vi "ASGS_device_serial_mode.vi"() -> ()   [LabVIEW 2017]
uses:
  <vilib>/Utility/file.llb/Read Delimited Spreadsheet (DBL).vi
  <vilib>/Instr/_visa.llb/VISA Configure Serial Port (Instr).vi
panel:
  in  "Match Pressure":bool
  out "While loop":dbl
  in  "Flow C. Baud Rate":u32=9600
  in  "Flow Controller Port":refnum<visa-resource-name>
  out "Constriction Percent":dbl
  out "Desired Subglottal Pressure":dbl
  in  "Number of Tests":dbl
  in  "SGS Device Port":refnum<visa-resource-name>
  in  "SGS Device Baud Rate":u32=9600
  out "Current Constriction":dbl
  # "SGS DEVICE CONTROL"
  # "USB Control"
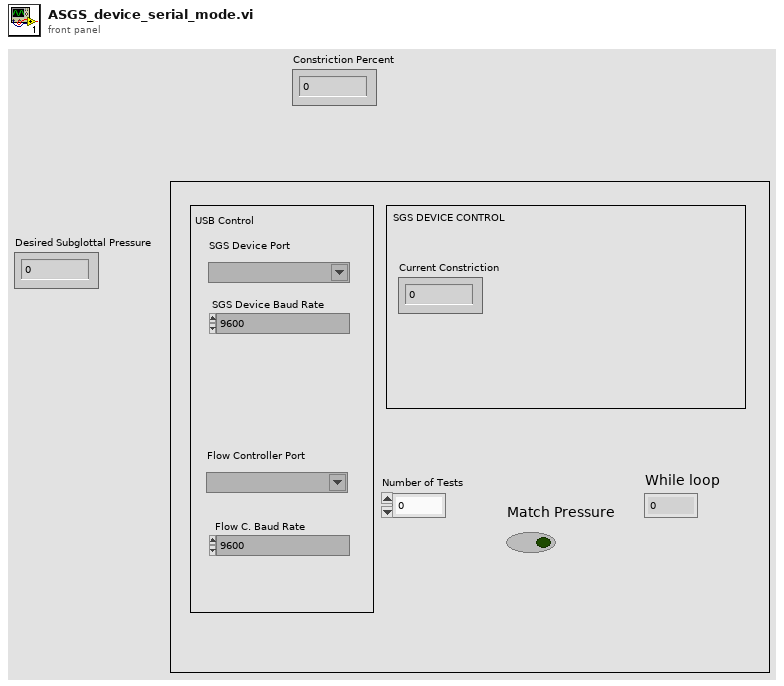
[diagram p1: front panel]
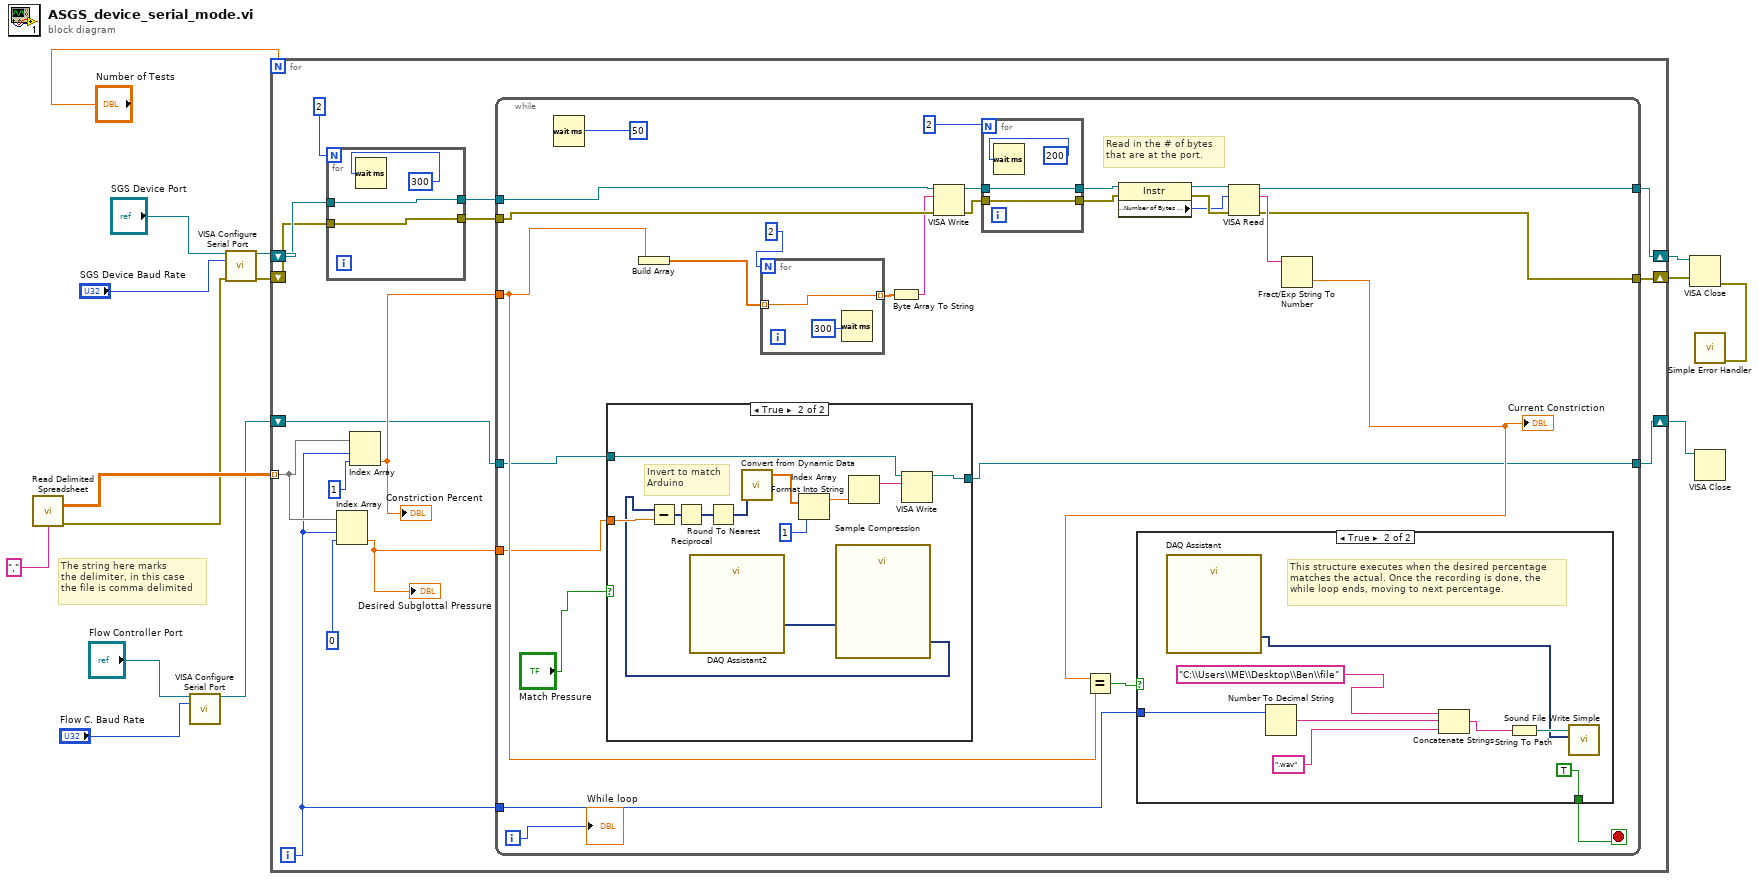
[diagram p0: block diagram]
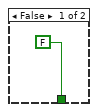
[diagram p3: hidden frame]
diagram:
  # "The string here marks\nthe delimiter, in this case\nthe file is comma delimited"
  n1 = call-poly <vilib>:"Read Delimited Spreadsheet.vi"("delimiter (\\t)"=",") -> ("all rows"=w8:dbl[][], "error out"=w6:errorcluster)  [unwired: 9 in, 4 out]
  n2 = call-poly "VISA Configure Serial Port"("VISA resource name"="Flow Controller Port", "baud rate (9600)"="Flow C. Baud Rate") -> ("VISA resource name out"=w2:refnum<visa-resource-name>)  [unwired: 12 in, 1 out]
  n3 = call-poly "VISA Configure Serial Port"("VISA resource name"="SGS Device Port", "baud rate (9600)"="SGS Device Baud Rate", "error in (no error)"=w6) -> ("VISA resource name out"=w10:refnum<visa-resource-name>, "error out"=w9:errorcluster)  [unwired: 11 in]
  n4 = for {
    N: "Number of Tests" -> [_]
    shift-right: [w23] -> w14
    shift-left: w10 -> [w20]
    shift-right: [w24] -> w15
    shift-left: w9 -> [w19]
    tunnel: w8 -> [w30] mode=indexing
    shift-right: [w22] -> w1
    shift-left: w2 -> [w25]
    i -> [w26]
    n5 = for {
      N: 2 -> [_]
      tunnel: [w33] -> w21
      tunnel: w20 -> [w33]
      tunnel: w19 -> [w32]
      tunnel: [w32] -> w18
      n6 = Wait (ms)(milliseconds to wait=300) -> ()  [unwired: 1 out]
    }
    n7 = Index Array(array=w30, index #1=w26, index #2=0) -> (element #2=w16:dbl)  [unwired: 1 out]
    "Desired Subglottal Pressure" <- w16
    n8 = Index Array(array=w30, index #1=w26, index #2=1) -> (element #2=w27:dbl)  [unwired: 1 out]
    "Constriction Percent" <- w27
    n9 = while {
      tunnel: w27 -> [w58]
      tunnel: w26 -> [w60]
      tunnel: w21 -> [w52]
      tunnel: w18 -> [w53]
      tunnel: [w48] -> w24
      tunnel: w25 -> [w37]
      tunnel: [w36] -> w22
      tunnel: [w47] -> w23
      tunnel: w16 -> [w35]
      i -> [w55]
      stop <- w56 stop-if-true
      # "Read in the # of bytes \nthat are at the port."
      n10 = Wait (ms)(milliseconds to wait=u32 50 ("millisecond timer value")) -> ()  [unwired: 1 out]
      n11 = case shown="True" "Match Pressure" {
        tunnel: w35 -> [_ w69]
        tunnel: [w62 w67] -> w36
        tunnel: w37 -> [w62 w66]
        frame False {
        }
        frame True {
          # "Invert to match\nArduino"
          n12 = call "DAQ Assistant2"() -> ("data"=w74:dynamicdata)  [unwired: 17 in, 2 out]
          n13 = call "Sample Compression"("Signals"=w74) -> ("Mean"=w68:dynamicdata)  [unwired: 8 in, 2 out]
          n14 = Subtract(x=w68, y=w69) -> (x-y=w65:dynamicdata)
          n15 = Reciprocal(x=w65) -> (1/x=w64:dynamicdata)
          n16 = Round To Nearest(number=w64) -> (nearest integer value=w63:dynamicdata)
          n17 = call "Convert from Dynamic Data"("Dynamic Data Type"=w63) -> ("Array"=w71:dbl[])  [unwired: 3 in]
          n18 = Index Array(array=w71, index=1) -> (element=w72:dbl)
          n19 = Format Into String(w72) -> (resulting string=w73:string)  [unwired: 3 in, 1 out]
          n20 = VISA Write(VISA resource name=w66, write buffer=w73) -> (VISA resource name out=w67:refnum<visa-resource-name>)  [unwired: 1 in, 2 out]
        }
      }
      n21 = Build Array(w58) -> (w45:dbl[])
      n22 = for {
        N: 2 -> [_]
        tunnel: [w79] -> w46 mode=indexing
        tunnel: w45 -> [w79] mode=indexing
        n23 = Wait (ms)(milliseconds to wait=300) -> ()  [unwired: 1 out]
      }
      n24 = Byte Array To String(unsigned byte array=w46) -> (string=w44:string)
      n25 = VISA Write(VISA resource name=w52, write buffer=w44, error in (no error)=w53) -> (VISA resource name out=w42:refnum<visa-resource-name>, error out=w40:errorcluster)  [unwired: 1 out]
      n26 = for {
        N: 2 -> [_]
        tunnel: [w77] -> w43
        tunnel: w42 -> [w77]
        tunnel: [w76] -> w41
        tunnel: w40 -> [w76]
        n27 = Wait (ms)(milliseconds to wait=200) -> ()  [unwired: 1 out]
      }
      n28 = property class="Instr"(reference=w43, error in=w41) -> (reference out=w51:refnum<visa-resource-name>, error out=w50:errorcluster, "Serial Settings:Number of Bytes at Serial Port"=w49:u32)
      n29 = VISA Read(VISA resource name=w51, byte count=w49, error in (no error)=w50) -> (VISA resource name out=w47:refnum<visa-resource-name>, read buffer=w54:string, error out=w48:errorcluster)  [unwired: 1 out]
      n30 = Fract/Exp String To Number(string=w54) -> (number=w57:dbl)  [unwired: 3 in, 1 out]
      "Current Constriction" <- w57
      n31 = Equal?(x=w57, y=w58) -> (x = y?=w59:bool)
      n32 = case shown="True" w59 {
        tunnel: w60 -> [_ w88]
        tunnel: [FALSE TRUE] -> w56
        frame False {
        }
        frame True {
          # "This structure executes when the desired percentage\nmatches the actual. Once the recording is done, the\nwhile loop ends, moving to next percentage."
          n33 = call "DAQ Assistant"() -> ("data"=w82:dynamicdata)  [unwired: 17 in, 2 out]
          n34 = Number To Decimal String(number=w88) -> (decimal integer string=w86:string)  [unwired: 1 in]
          n35 = Concatenate Strings("C:\\Users\\ME\\Desktop\\Ben\\file", w86, ".wav") -> (w84:string)
          n36 = String To Path(string=w84) -> (path=w83:path)
          n37 = call <vilib>:"Sound File Write Simple.vi"("data"=w82, "path"=w83) -> ()  [unwired: 8 in, 2 out]
        }
      }
      "While loop" <- w55
    }
  }
  n38 = VISA Close(VISA resource name=w14, error in (no error)=w15) -> (error out=w13:errorcluster)
  n39 = call <vilib>:"Simple Error Handler.vi"("error in (no error)"=w13) -> ()  [unwired: 4 in, 5 out]
  n40 = VISA Close(VISA resource name=w1) -> ()  [unwired: 1 in, 1 out]
